vi "Focus Track Stack.vi"(7 "Filter Etch Figures":bool, 8 "error in (no error)":errorcluster, 9 "Grayscale?":bool, 10 "Kernel Size":i32, 11 "Path":path) -> (0 "error out":errorcluster, 2 "Height Map":T1(plugin-control), 3 "Image":T1(plugin-control))   [LabVIEW 2013]
uses:
  <vilib>/vision/NI_Vision_Development_Module.lvlib
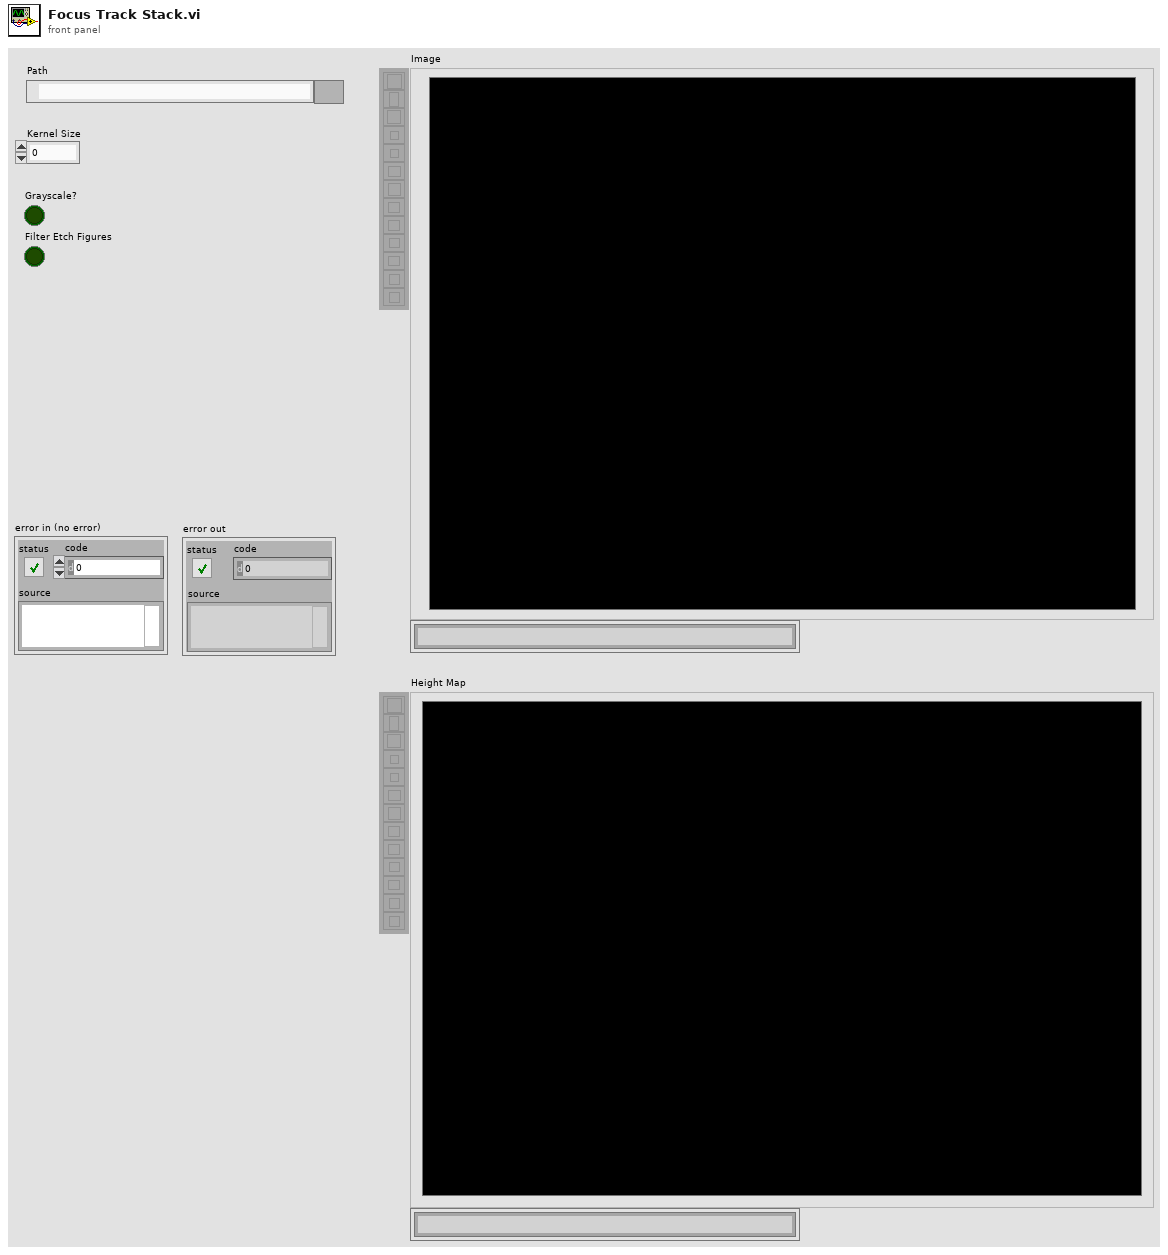
[diagram p1: front panel]
types:
  T1 = typedef "IMAQ Image.ctl" = refnum<image>
  T2 = typedef "Image Type" = u32
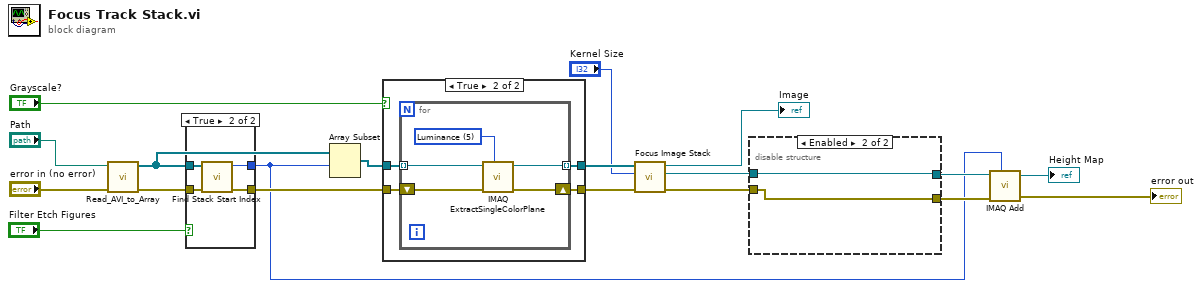
[diagram p0: block diagram]
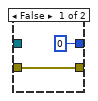
[diagram p2: hidden frame]
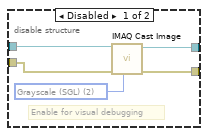
[diagram p3: hidden frame]
diagram:
  n1 = call "Read_AVI_to_Array.vi"("Error in (no error)"="error in (no error)", "AVI Path"="Path") -> ("Error out"=w10:errorcluster, "Image Array"=w9:T1[])  [unwired: 7 in, 1 out]
  n2 = case shown="True" "Filter Etch Figures" {
    tunnel: w10 -> [w21 w25]
    tunnel: w9 -> [_ w24]
    tunnel: [w21 w23] -> w8
    tunnel: [0 ("Start Index") w22] -> w2
    frame False {
    }
    frame True {
      n3 = call "Find Stack Start Index.vi"("error in (no error)"=w25, "Image Array"=w24) -> ("error out"=w23:errorcluster, "Start Index"=w22:i32)  [unwired: 8 in]
    }
  }
  n4 = Array Subset(array=w9, index=w2) -> (w11:T1[])  [unwired: 1 in]
  n5 = case shown="True" "Grayscale?" {
    tunnel: w8 -> [w26 w31]
    tunnel: w11 -> [w27 w30]
    tunnel: [w27 w29] -> w16
    tunnel: [w26 w28] -> w15
    frame False {
    }
    frame True {
      n6 = for {
        shift-right: [w34] -> w28
        shift-left: w31 -> [w36]
        tunnel: w30 -> [w35] mode=indexing
        tunnel: [w33] -> w29 mode=indexing
        w32 = 5 items=["Red", "Green", "Blue", "Hue", "Saturation", "Luminance", "Value", "Intensity"] ("Color Plane")
        n7 = call "IMAQ ExtractSingleColorPlane"("Color Plane"=w32, "error in (no error)"=w36, "Image Src"=w35) -> ("error out"=w34:errorcluster, "Image Dst Out"=w33:T1)  [unwired: 7 in]
      }
    }
  }
  n8 = call "Focus Image Stack.vi"("error in (no error)"=w15, "Kernel Size"="Kernel Size", "Image Stack"=w16) -> ("error out"=w5:errorcluster, "Height Map"=w12:T1, "Focused Image"=→"Image":T1)  [unwired: 6 in]
  n9 = disable-structure shown="Enabled" {
    disable-tunnel: w12 -> [w41 w43]
    disable-tunnel: [w40 w43] -> w7
    disable-tunnel: w5 -> [w38 w42]
    disable-tunnel: [w37 w42] -> w4
    frame Disabled {
      w39 = T2 2 items=["Grayscale (U8)", "Grayscale (I16)", "Grayscale (SGL)", "Complex (CSG)", "RGB (U32)", "HSL (U32)", "RGB (U64)", "Grayscale (U16)"] ("Image Type")
      # "Enable for visual debugging"
      n10 = call "IMAQ Cast Image"("Image Type"=w39, "error in (no error)"=w38, "Image Src"=w41) -> ("error out"=w37:errorcluster, "Image Dst Out"=w40:T1)  [unwired: 3 in, 4 out]
    }
    frame Enabled {
    }
  }
  n11 = call "IMAQ Add"("Image Src A"=w7, "Constant"=w2, "error in (no error)"=w4) -> ("Image Dst Out"=→"Height Map":T1, "error out"=→"error out":errorcluster)  [unwired: 4 in]
